vi "Digital Write - Challenge.vi"() -> ()   [LabVIEW 2009]
uses:
  <vilib>/DAQmx/create/channels.llb/DAQmx Create Channel (DO-Digital Output).vi
  <vilib>/DAQmx/write.llb/DAQmx Write (Digital 1D Bool 1Chan 1Samp).vi
panel:
  in  "lines":tag="Dev1/port0/line0:7"
  in  "data":bool[](array[boolean])=[TRUE, TRUE, TRUE, TRUE, TRUE, TRUE, TRUE, TRUE]
  in  "stop":bool
  # "CHALLENGE\nModify the VI so that the boolean array control will better reflect the actual orientation\nof the LEDs on the BNC-2120.\n\n1. Added the Reverse 1D Array function to block diagram.\n2. Removed the Index Display from the Visible Items of the data boolean array control.\n3. Added labels."
  # "DIO7"
  # "DIO6"
  # "DIO5"
  # "DIO4"
  # "DIO3"
  # "DIO2"
  # "DIO1"
  # "DIO0"
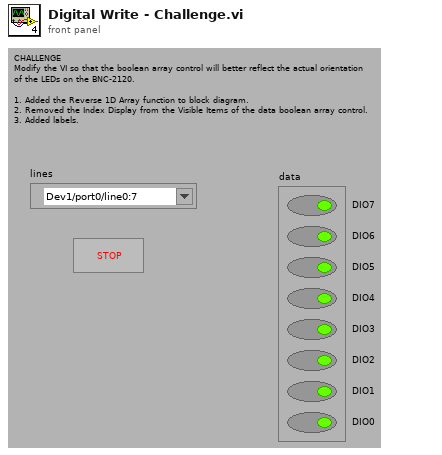
[diagram p1: front panel]
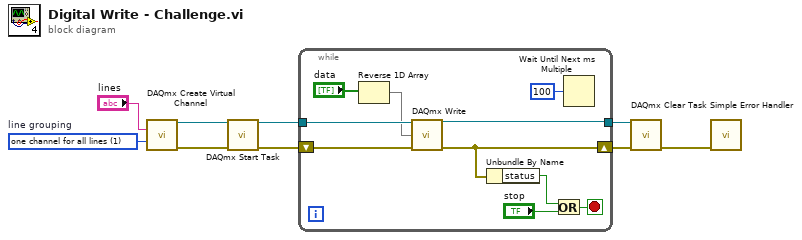
[diagram p0: block diagram]
diagram:
  w2 = 1 items=["one channel for each line", "one channel for all lines"]  # line grouping
  n1 = call-poly <vilib>:"DAQmx Create Virtual Channel.vi"("lines"="lines", "line grouping"=w2) -> ("task out"=w9:refnum<k21>, "error out"=w6:errorcluster)  [unwired: 12 in]
  n2 = call <vilib>:"DAQmx Start Task.vi"("task/channels in"=w9, "error in"=w6) -> ("task out"=w8:refnum<k21>, "error out"=w5:errorcluster)  [unwired: 12 in]
  n3 = while {
    tunnel: w8 -> [w19]
    tunnel: [w18] -> w7
    shift-right: [w16] -> w4
    shift-left: w5 -> [w17]
    stop <- w13 stop-if-true
    n4 = Reverse 1D Array(array="data") -> (reversed array=w10:bool[])
    n5 = call-poly <vilib>:"DAQmx Write.vi"("task/channels in"=w19, "data"=w10, "error in"=w17) -> ("task out"=w18:refnum<k21>, "error out"=w16:errorcluster)  [unwired: 10 in, 1 out]
    n6 = Unbundle By Name "Unbundle By Name"(w16) -> ("status"=w15:bool)
    n7 = Or(x=w15, y="stop") -> (x .or. y?=w13:bool)
    n8 = Wait Until Next ms Multiple(millisecond multiple=u32 100) -> ()  [unwired: 1 out]
  }
  n9 = call <vilib>:"DAQmx Clear Task.vi"("task in"=w7, "error in"=w4) -> ("error out"=w3:errorcluster)  [unwired: 13 in]
  n10 = call <vilib>:"Simple Error Handler.vi"("error in (no error)"=w3) -> ()  [unwired: 4 in, 5 out]
